vi "LSX Get Status Axis.vi"(8 "error in (no error)":errorcluster, 9 "lMaxLen":i32, 10 "pcStatusAxisStr":string, 11 "lLSID":i32) -> (0 "error out":errorcluster, 2 "pcStatusAxisStr out":string, 3 "function return":i32)   [LabVIEW 2018, in "Tango.lvlib"]
doc: "TANGOAPI int TANGOCALL LSX_GetStatusAxis (int lLSID, char *pcStatusAxisStr, int lMaxLen);"
uses:
  Tango.lvlib
  SubVIs/Tango_DLL.dll
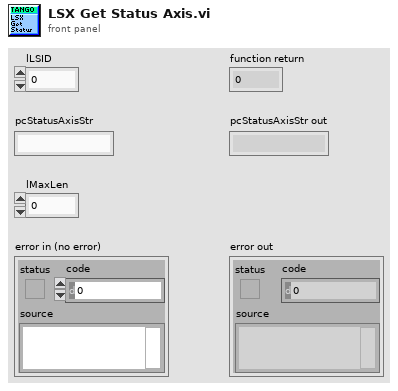
[diagram p1: front panel]
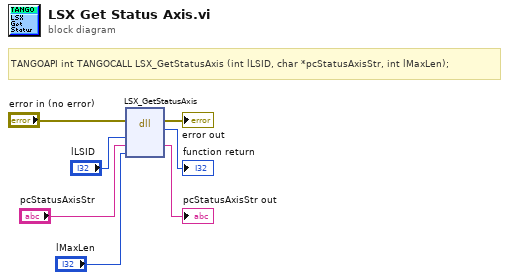
[diagram p0: block diagram]
diagram:
  # "TANGOAPI int TANGOCALL LSX_GetStatusAxis (int lLSID, char *pcStatusAxisStr, int lMaxLen);"
  n1 = dll-call lib="C:/Users/Familie/Documents/LabviewIX81/lib/TANGO Stage/SubVIs/Tango_DLL.*" fn="LSX_GetStatusAxis"(error in="error in (no error)", "lLSID"="lLSID", "pcStatusAxisStr"="pcStatusAxisStr", "lMaxLen"="lMaxLen") -> (error out=→"error out":errorcluster, →"function return":i32, "pcStatusAxisStr"=→"pcStatusAxisStr out":string)  [unwired: 4 in, 1 out]
